vi "TLB Native Dynamic Events ver 0.09.vi"() -> ()   [LabVIEW 2018]
uses:
  Labview Training Phase 2/Enum Controls/States for Action Engine.ctl
  Type def/TLB event states.ctl
  Type def/TLB MHL States.ctl
  <vilib>/Studica/Studica Toolkit/Background/I2C Channel.ctl
  <vilib>/myRIO/Common/Instrument Driver Framework/myRIO v1.0/AI/typedefs/AI Channels Enum.ctl
  <vilib>/myRIO/Common/Instrument Driver Framework/myRIO v1.0/AI/typedefs/AI Channels List.ctl
  Type def/Type def.ctl
  <vilib>/addons/control/pid/NI_PID_pid.lvlib
  Underlying VI's/Webcam FGV Low level ver/State control.ctl
  <vilib>/userdefined/High Color/IMAQdx.ctl
  <vilib>/Studica/Studica Toolkit/NavX/NavX.lvlib
  <vilib>/addons/control/pid/pid.llb/PID (DBL).vi
  Underlying VI's/Movement control (archived)/Motor Control/States for motor control.ctl
  <vilib>/NI_Real-Time Target Support.lvlib
panel:
  out "Arduino Data":T1
  in  "STOP TASK":bool
  out "Waveform Chart 2":dbl(graph)
  in  "Select task":i8
  in  "OK Button":bool
  out "Yaw":dbl
  out "Speed and distance cluster":T2
  out "Decision":i8
  in  "STOP":bool
  out "error out":errorcluster
  out "Object detection count":T3
  out "Camera error":errorcluster
  out "element":T4
  out "Action Queue Items":i32
  out "State Logic Queue Items":i32
  out "Action Queues items":string[](array[string])=["Hardware reset", "Software reset", ""]
  out "State logic":T5=enum."Task 2"
  out "Action State":string
  # "TLB FRAMEWORK STATUS"
  # "Camera Status Loop"
  # "Test Programme written by Calvin Loke    Dated: 28 Aug 2019\nTest Programme revised by Dr Alex See   Dated 30 Aug 2019\n\nProgramme version:   TLB Native Dynamic Events ver 0.04b.vi"
  # "Motor Control Loop"
  # "NAVX Control Loop"
  # "Blackhawk status"
  # "System Health Status Update"
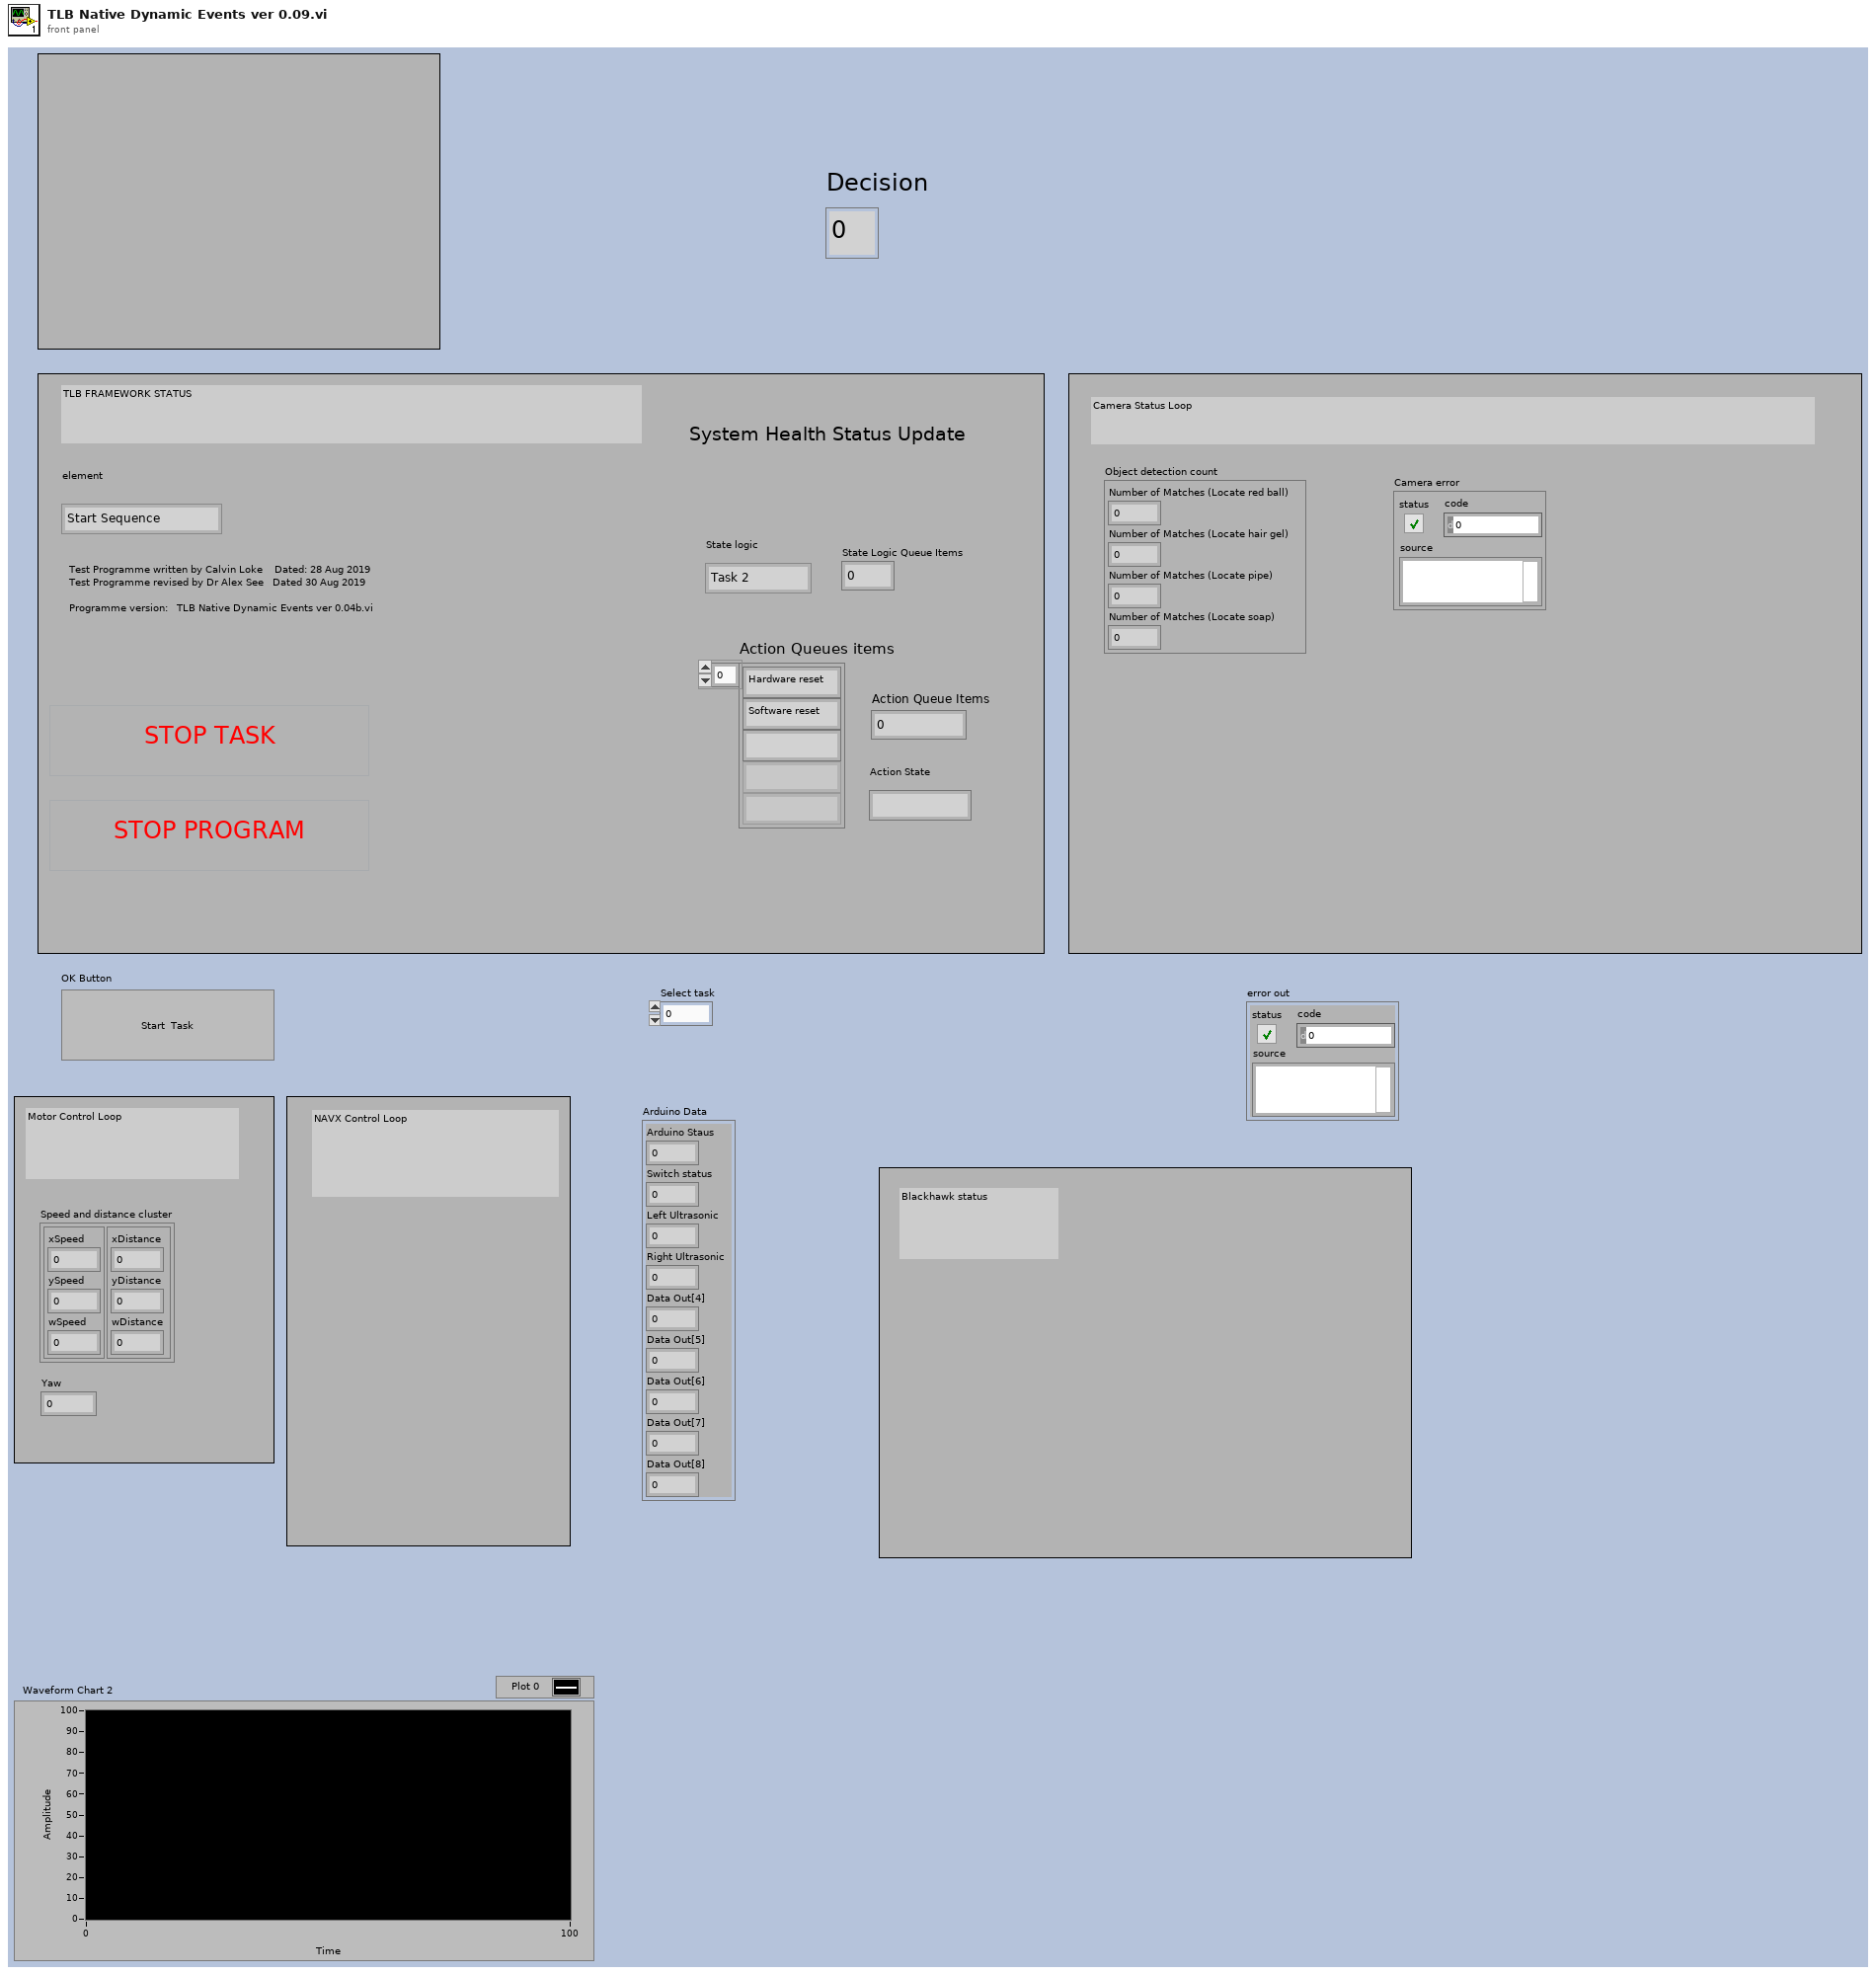
[diagram p1: front panel]
types:
  T1 = cluster{"Arduino Staus":u8, "Switch status":u8, "Left Ultrasonic":u8, "Right Ultrasonic":u8, "Data Out[4]":u8, "Data Out[5]":u8, "Data Out[6]":u8, "Data Out[7]":u8, "Data Out[8]":u8}
  T2 = cluster{cluster{"xSpeed":dbl, "ySpeed":dbl, "wSpeed":dbl}, cluster{"xDistance":dbl, "yDistance":dbl, "wDistance":dbl}}
  T3 = cluster{"Number of Matches (Locate red ball)":i32, "Number of Matches (Locate hair gel)":i32, "Number of Matches (Locate pipe)":i32, "Number of Matches (Locate soap)":i32}
  T4 = typedef "TLB event states.ctl" = enum16{"Start Sequence", "Exit", "Start Task 1", "Start Task 2", "Start Task 3", "Start Task 4", "Camera vision", "Wall follow mode", "Idle", "Start Drive Straight"}
  T5 = typedef "TLB MHL States.ctl" = enum16{"None", "Startup", "Idle", "Processing", "Shutdown", "Reset", "Task 1", "Task 2", "Task 3", "Task 4", "Task 4a", "Task 4b", "Task 4c", "Task 4d", "Task 4e", "Task 4f", "Task 4g", "Task 4h", "Acquire image", "Wall follow mode", "Autodrive", "Autodrive a"}
  T6 = typedef "States for motor control.ctl" = enum16{"LAST STATE", "STOP", "FORWARD", "BACKWARD", "LEFT", "RIGHT", "RCW", "ACW", "INIT", "RESET ENCODERS"}
  T7 = typedef "States for Action Engine.ctl" = enum16{"Initialize", "Write", "Read"}
  T8 = typedef "Type def.ctl" = cluster{"Front Ultrasonic Obstruct":bool, "Left Ultrasonic Obstruct":bool, "Right Ultrasonic Obstruct ":bool}
  T9 = typedef "I2C Channel.ctl" = enum16{"Not Connected", "A", "B"}
  T10 = enum16{"LAST STATE", "STOP", "FORWARD", "BACKWARD", "LEFT", "RIGHT", "RCW", "ACW", "INIT", "RESET ENCODERS"}
  T11 = cluster{"proportional gain (Kc)":dbl, "integral time (Ti, min)":dbl, "derivative time (Td, min)":dbl}
  T12 = typedef "State control.ctl" = enum16{"Initialise", "Start camera", "Continuous Acquisition ", "Stop camera", "Dispose all"}
  T13 = typedef "IMAQdx.ctl" = refnum<k21>
  T14 = cluster{"Arduino Status":u8, "Task Selection":u8, "PING_A":u8, "PING_B":u8, "PING_C":u8, "PING_D":u8, "Compass Low Byte":u8, "Compass High Byte":u8, "Data Out[8]":u8}
  T15 = typedef "AI Channels List.ctl" = T16[]
  T16 = typedef "AI Channels Enum.ctl" = enum16{"Not Connected", "AudioIn/Left", "AudioIn/Right", "C/AI0", "C/AI1", "A/AI0", "A/AI1", "A/AI2", "A/AI3", "A/AI4", "A/AI5", "A/AI6", "A/AI7", "B/AI0", "B/AI1", "B/AI2", "B/AI3", "B/AI4", "B/AI5", "B/AI6", "B/AI7", "AI/AI0", "AI/AI1", "AI/AI2", "AI/AI3", "A/AI0 (DIFF)", "A/AI1 (DIFF)", "A/AI2 (DIFF)", "A/AI3 (DIFF)", "B/AI0 (DIFF)", "B/AI1 (DIFF)", "B/AI2 (DIFF)", "B/AI3 (DIFF)"}
  T17 = typedef "NI_Real-Time Target Support.lvlib/RT CPU Load.ctl" = cluster{"Total (%)":dbl, "Time Critical (%)":dbl, "Timed Structures (%)":dbl, "High (%)":dbl, "Above Normal (%)":dbl, "Normal (%)":dbl, "Background (%)":dbl, "Idle (%)":dbl, "ISR (%)":dbl}
  T18 = cluster{"I2C Ref Out":cluster{"I2C Channel":T9, "FPGA VI Reference Out":refnum<k20>}, "Connected":bool, "Slave Address (7-bit)":u8, "Registry":u8[]}
  T19 = typedef "IMAQ Image.ctl" = refnum<image>
  T20 = cluster{"CPU loads[0]":T17, "CPU loads[1]":T17, "CPU loads[2]":T17, "CPU loads[3]":T17, "CPU loads[4]":T17, "CPU loads[5]":T17, "CPU loads[6]":T17, "CPU loads[7]":T17, "CPU loads[8]":T17}
  T21 = cluster{"Yaw":dbl, "Roll":dbl, "Pitch":dbl, "Heading":dbl, "Fused Heading":dbl}
  T22 = cluster{"xDistance":dbl, "yDistance":dbl, "wDistance":dbl}
  T23 = cluster{"I2C Channel":T9, "FPGA VI Reference Out":refnum<k20>}
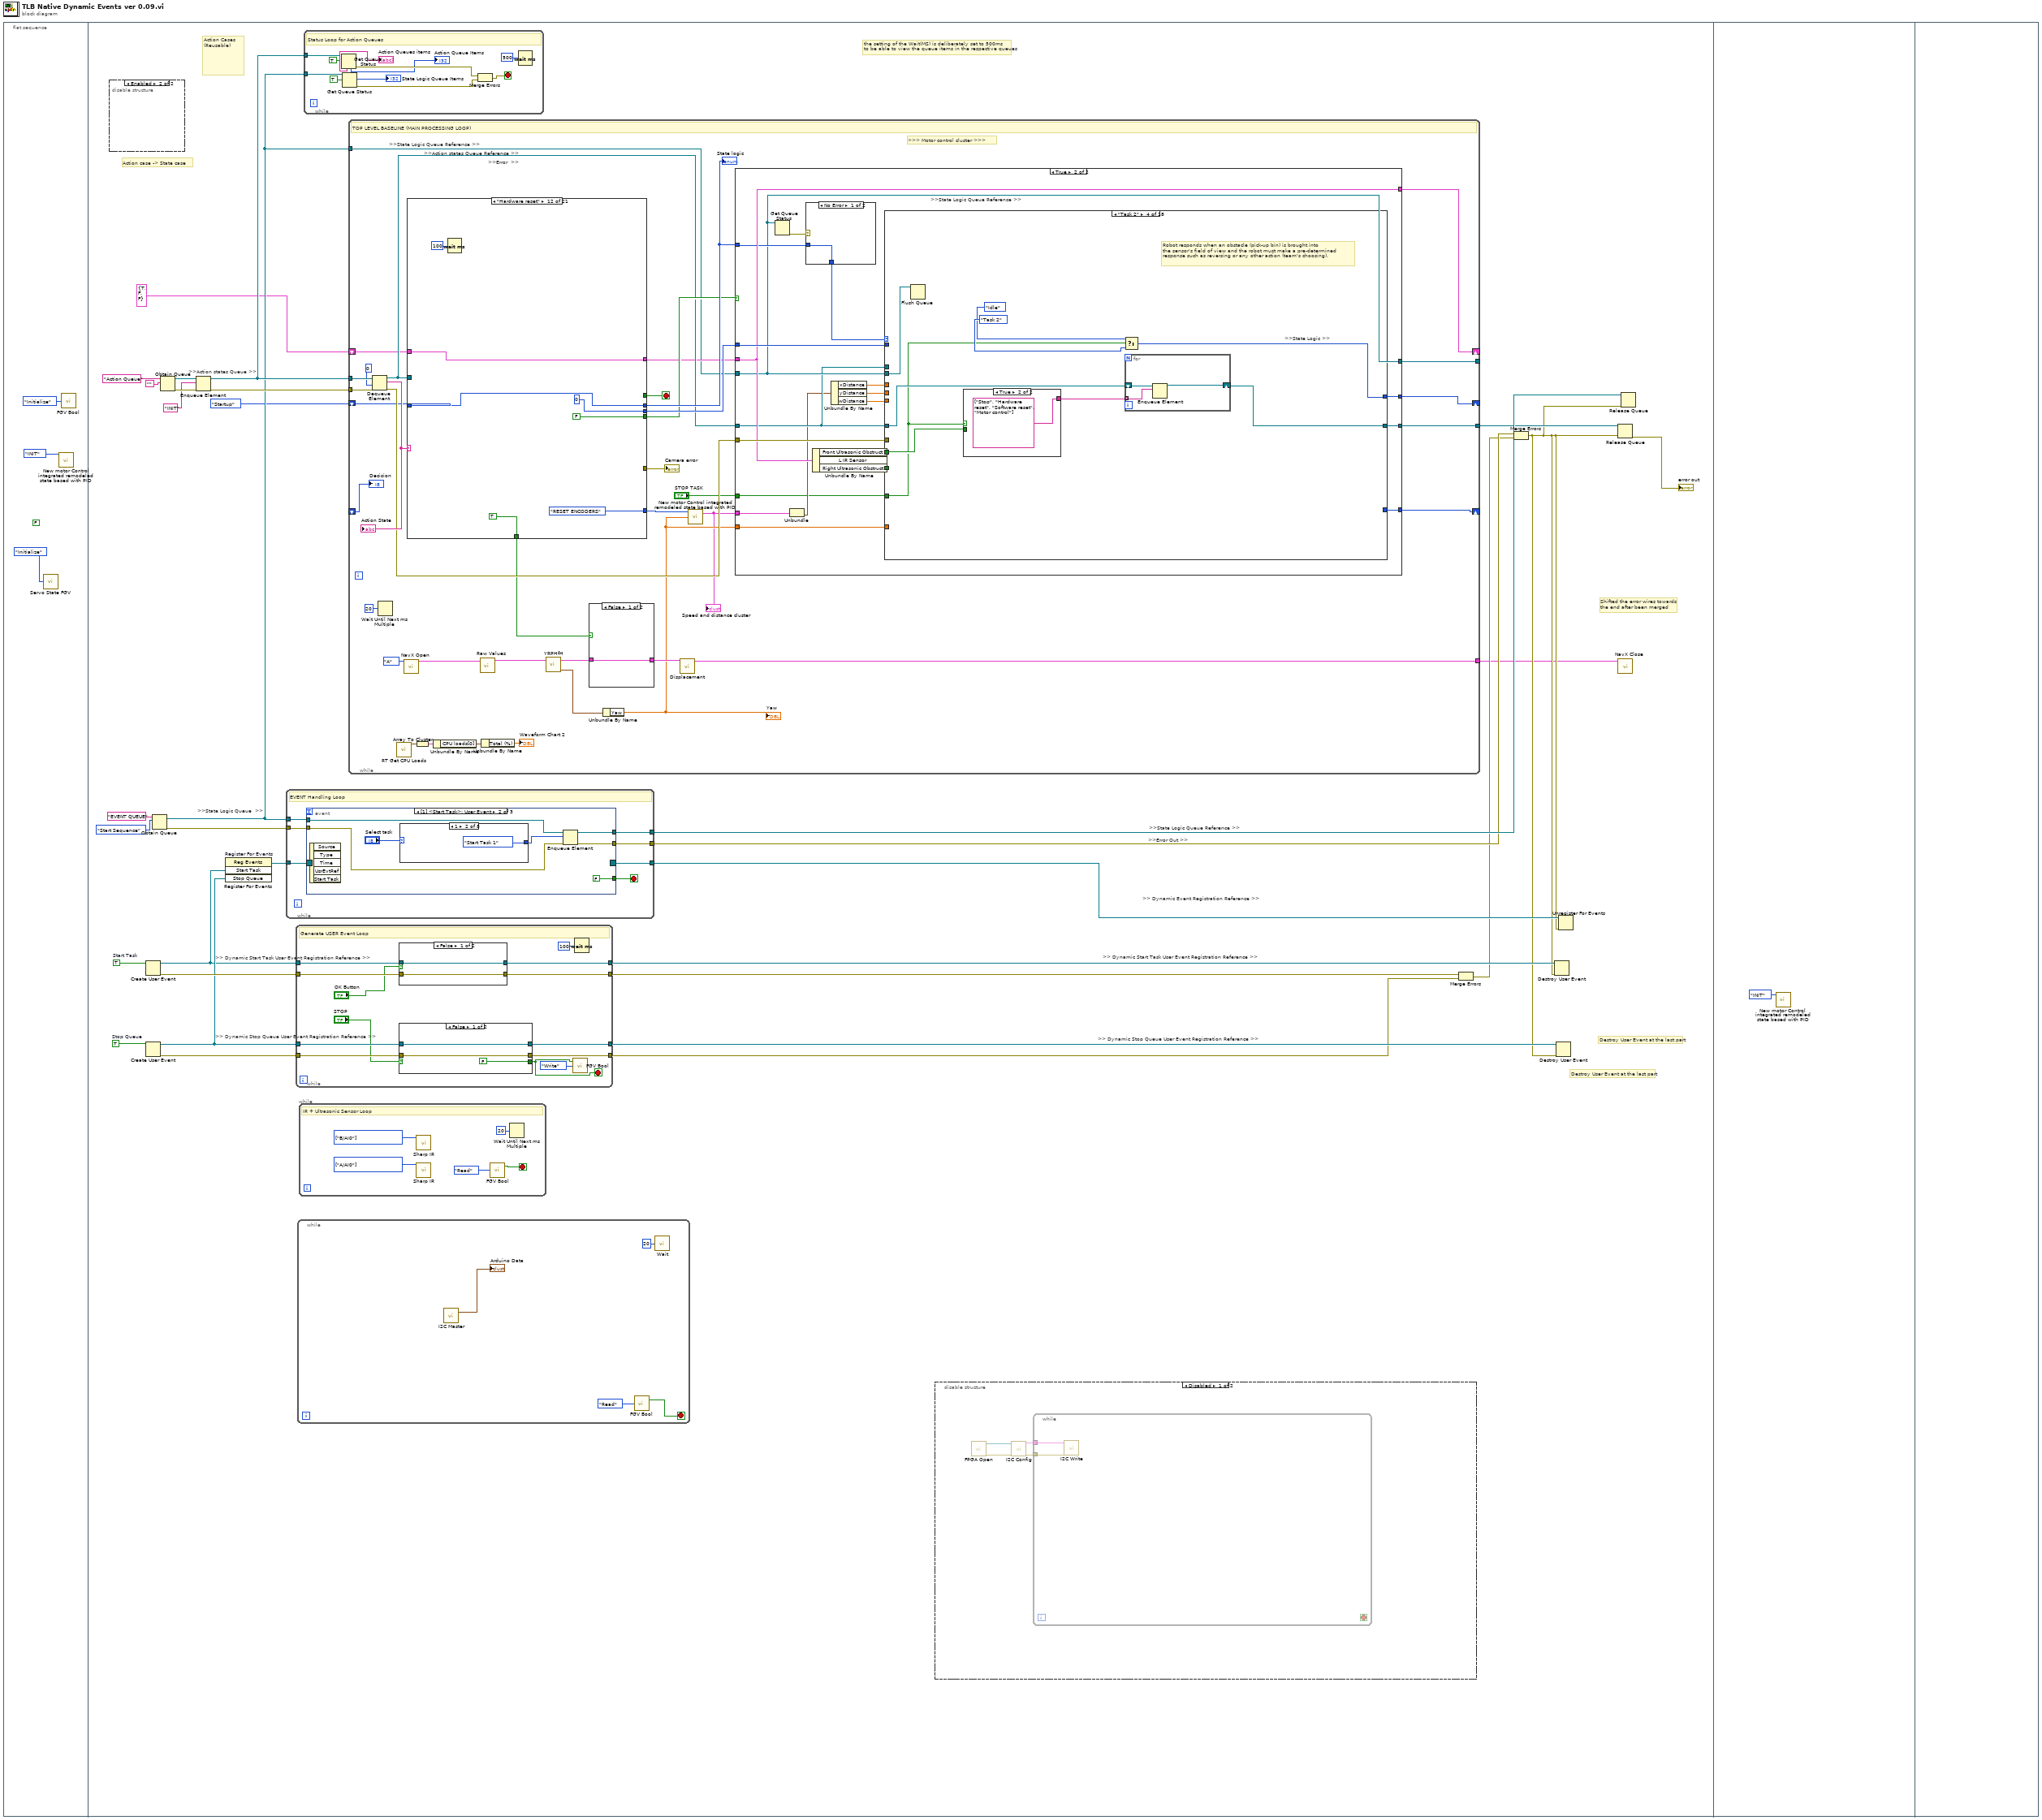
[diagram p0: block diagram]
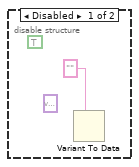
[diagram p3: hidden frame]
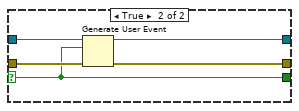
[diagram p4: hidden frame]
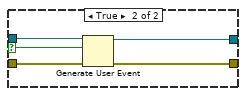
[diagram p5: hidden frame]
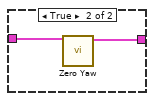
[diagram p6: hidden frame]
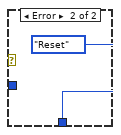
[diagram p8: hidden frame]
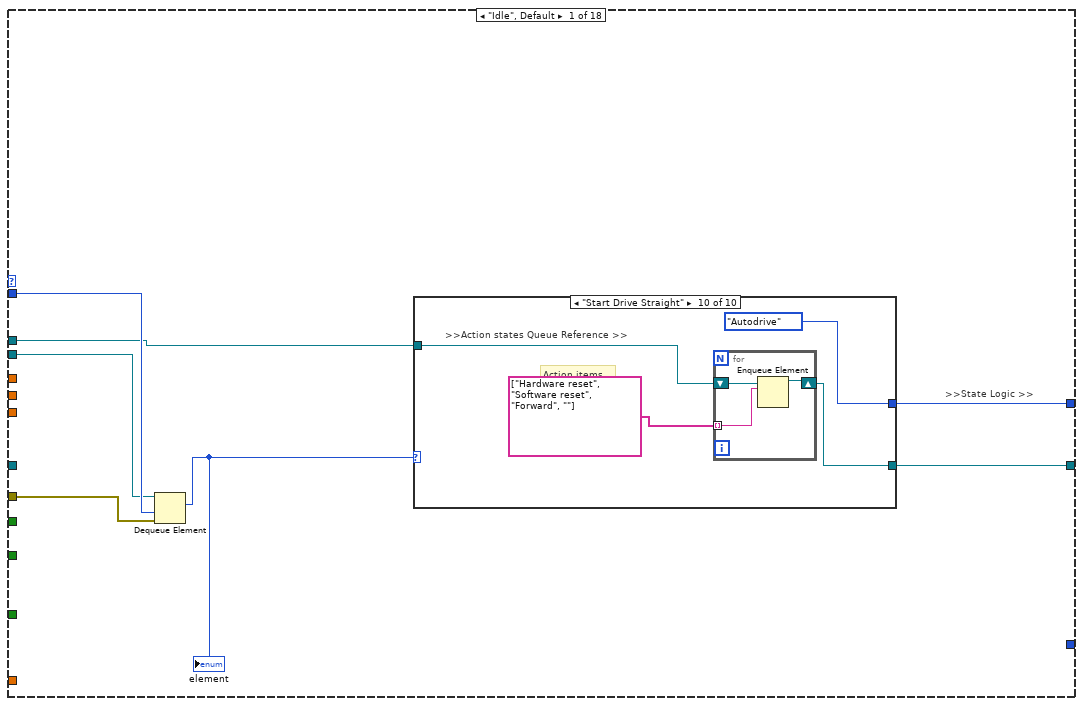
[diagram p9: hidden frame]
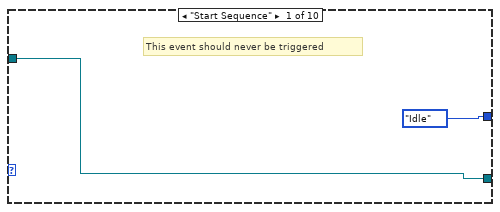
[diagram p10: hidden frame]
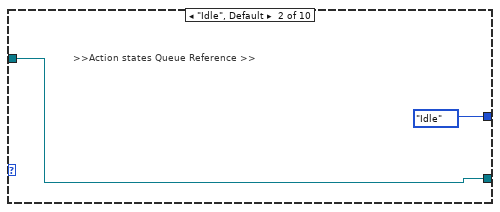
[diagram p11: hidden frame]
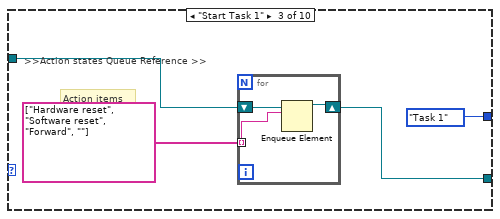
[diagram p12: hidden frame]
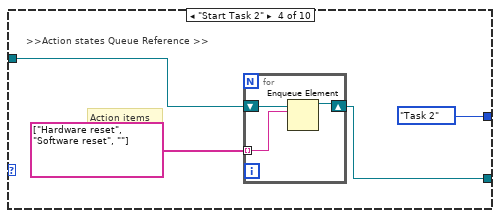
[diagram p13: hidden frame]
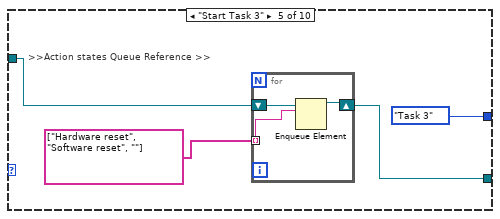
[diagram p14: hidden frame]
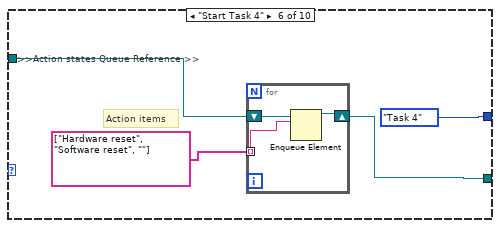
[diagram p15: hidden frame]
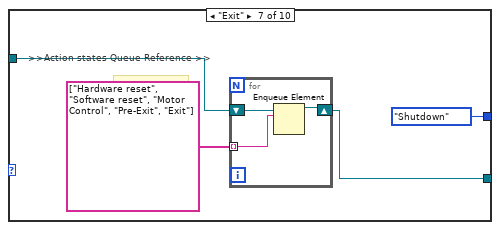
[diagram p16: hidden frame]
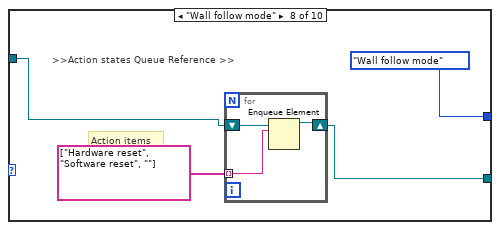
[diagram p17: hidden frame]
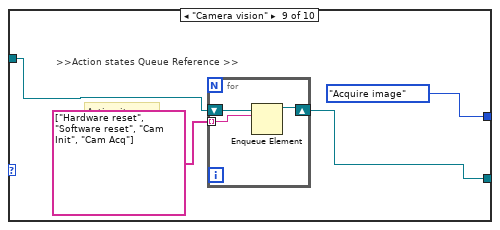
[diagram p18: hidden frame]
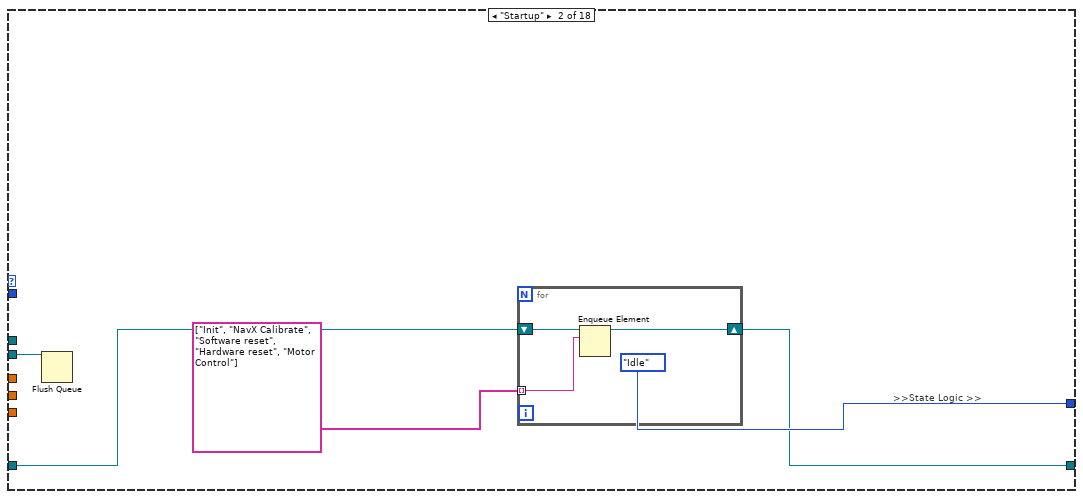
[diagram p19: hidden frame]
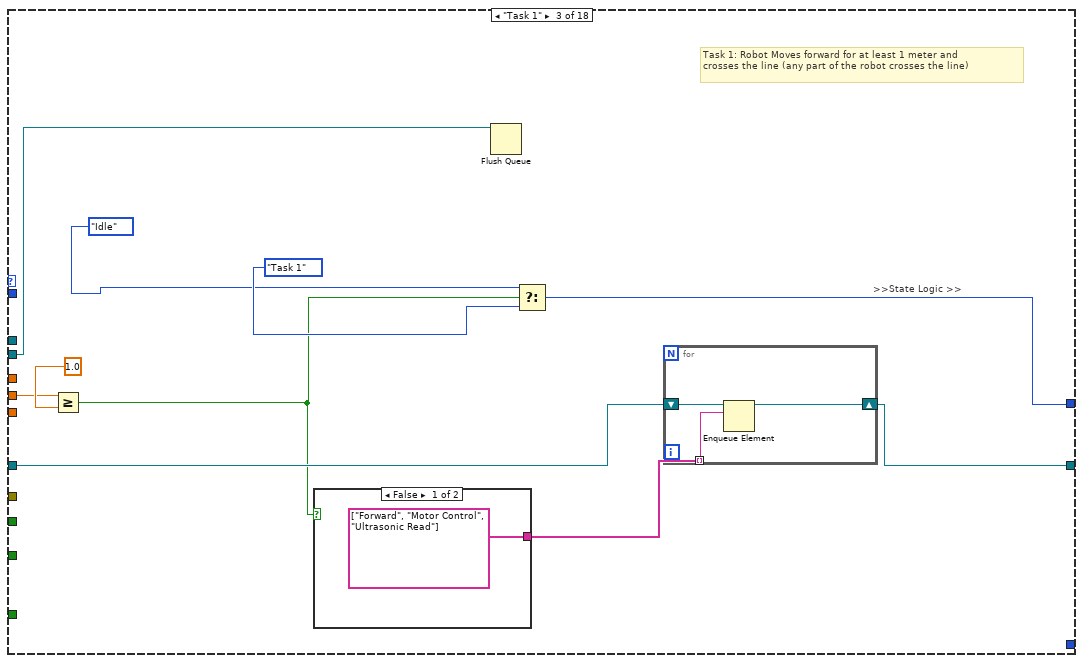
[diagram p20: hidden frame]
diagram:
  n1 = flat-sequence {
    frame #0 {
      (unwired) FALSE ("DIO 1")
      n2 = call "Servo State FGV.vi"("Init/Read/Write State"=States_for_Action_Engine."Initialize") -> ()  [unwired: 2 in, 2 out]
      n3 = call "New motor Control integrated remodeled state based with PID.vi"("States"=States_for_motor_control."INIT") -> ()  [unwired: 2 in, 2 out]
      n4 = call "FGV Bool.vi"("Init/Read/Write State"=States_for_Action_Engine."Initialize") -> ()  [unwired: 2 in, 2 out]
    }
    frame #1 {
      w35 = TRUE  # Stop Queue
      w34 = TRUE  # Start Task
      # "Action case -> State case"
      # "the setting of the Wait(MS) is deliberately set to 500ms\nto be able to view the queue items in the respective queues"
      # "Action Cases\n(Reusable)"
      # ">>Error Out >>"
      # ">> Dynamic Stop Queue User Event Registration Reference >>"
      # ">> Dynamic Start Task User Event Registration Reference >>"
      # ">> Dynamic Stop Queue User Event Registration Reference >>"
      # ">> Dynamic Start Task User Event Registration Reference >>"
      # ">> Dynamic Event Registration Reference >>"
      # ">>Action states Queue >>"
      # ">>State Logic Queue  >>"
      # ">>State Logic Queue Reference >>"
      # "Destroy User Event at the last part"
      # "Destroy User Event at the last part"
      # "Shifted the error wires towards\nthe end after been merged"
      n5 = disable-structure shown="Enabled" {
        frame Disabled {
          (unwired) variant
          (unwired) TRUE
          n6 = Variant To Data(type="") -> ()  [unwired: 2 in, 2 out]
        }
        frame Enabled {
        }
      }
      n7 = Create User Event(user event datatype=w34) -> (user event=w26:refnum<user-event>, error out=w31:errorcluster)  [unwired: 1 in]
      n8 = Create User Event(user event datatype=w35) -> (user event=w27:refnum<user-event>, error out=w30:errorcluster)  [unwired: 1 in]
      n9 = Obtain Queue(name (unnamed)="EVENT QUEUE", element data type=TLB_event_states."Start Sequence" ("Enum")) -> (queue out=w11:refnum<queue>, error out=w17:errorcluster)  [unwired: 3 in, 1 out]
      n10 = Obtain Queue(name (unnamed)="Action Queue", element data type="") -> (queue out=w20:refnum<queue>, error out=w16:errorcluster)  [unwired: 3 in, 1 out]
      n11 = Enqueue Element(queue=w20, element="INIT", error in (no error)=w16) -> (queue out=w12:refnum<queue>, error out=w15:errorcluster)  [unwired: 1 in, 1 out]
      n12 = register-events "Register For Events"(w26, w27) -> (reference out=w25:refnum<event-registration>)  [unwired: 2 in, 1 out]
      n13 = while {
        tunnel: w25 -> [w592]
        tunnel: [w591] -> w24
        tunnel: w11 -> [w589]
        tunnel: [w588] -> w23
        tunnel: w17 -> [w587]
        tunnel: [w586] -> w14
        stop <- w590 stop-if-true
        # "EVENT Handling Loop"
        n14 = event shown="[1] <Start Task>: User Event" {
          selector: w592 -> [_ _ _]
          dyn-events: [_ _ _] -> w591
          timeout: _ -> [_ _ _]
          tunnel: [FALSE FALSE w619] -> w590
          tunnel: w589 -> [w597 w604 w617]
          tunnel: [w596 w603 w618] -> w588
          tunnel: w587 -> [w594 w602 w615]
          tunnel: [w593 w601 w614] -> w586
          event Timeout {
            n15 = event-data() -> ()  [unwired: 1 in, 3 out]
            n16 = Enqueue Element(queue=w597, element=TLB_event_states."Idle" ("Enum"), error in (no error)=w594) -> (queue out=w596:refnum<queue>, error out=w593:errorcluster)  [unwired: 1 in, 1 out]
          }
          event User Event {
            n17 = event-data() -> ()  [unwired: 1 in, 5 out]
            n18 = case shown="1" "Select task" {
              tunnel: [TLB_event_states."Idle" ("Enum") TLB_event_states."Start Task 1" ("Enum") TLB_event_states."Start Task 2" ("Enum") TLB_event_states."Start Task 3" ("Enum") TLB_event_states."Start Task 4" ("Enum") TLB_event_states."Wall follow mode" ("Enum") TLB_event_states."Camera vision" ("Enum") TLB_event_states."Start Drive Straight" ("Enum")] -> w600
              frame 0 {
              }
              frame 1 {
              }
              frame 2 {
              }
              frame 3, Default {
              }
              frame 4 {
              }
              frame 5 {
              }
              frame 6 {
              }
              frame 7 {
              }
            }
            n19 = Enqueue Element(queue=w604, element=w600, error in (no error)=w602) -> (queue out=w603:refnum<queue>, error out=w601:errorcluster)  [unwired: 1 in, 1 out]
          }
          event User Event {
            n20 = event-data() -> ("Stop Queue"=w619:bool)  [unwired: 1 in, 4 out]
            n21 = Enqueue Element At Opposite End(queue=w617, element=TLB_event_states."Exit" ("Enum"), error in (no error)=w615) -> (queue out=w618:refnum<queue>, error out=w614:errorcluster)  [unwired: 1 in, 1 out]
          }
        }
      }
      n22 = while {
        tunnel: w26 -> [w69]
        tunnel: w27 -> [w68]
        tunnel: [w67] -> w33
        tunnel: [w66] -> w32
        tunnel: w31 -> [w65]
        tunnel: [w64] -> w29
        tunnel: w30 -> [w63]
        tunnel: [w62] -> w28
        stop <- w60 stop-if-true
        # "Generate USER Event Loop"
        n23 = case shown="False" "OK Button" {
          selector: "OK Button" -> [_ w81]
          tunnel: w69 -> [w80 w85]
          tunnel: [w80 w84] -> w66
          tunnel: w65 -> [w79 w83]
          tunnel: [w79 w82] -> w64
          frame False {
          }
          frame True {
            n24 = Generate User Event(user event=w85, event data cluster=w81, error in=w83) -> (user event out=w84:refnum<user-event>, error out=w82:errorcluster)  [unwired: 1 in]
          }
        }
        n25 = case shown="False" "STOP" {
          selector: "STOP" -> [_ w74]
          tunnel: w68 -> [w73 w78]
          tunnel: [w73 w77] -> w67
          tunnel: w63 -> [w72 w76]
          tunnel: [w72 w75] -> w62
          tunnel: [FALSE w74] -> w60
          frame False {
          }
          frame True {
            n26 = Generate User Event(user event=w78, event data cluster=w74, error in=w76) -> (user event out=w77:refnum<user-event>, error out=w75:errorcluster)  [unwired: 1 in]
          }
        }
        n27 = call "FGV Bool.vi"("Init/Read/Write State"=States_for_Action_Engine."Write", "Input Node"=w60) -> ()  [unwired: 1 in, 2 out]
        n28 = Wait (ms)(milliseconds to wait=u32 100) -> ()  [unwired: 1 out]
      }
      n29 = while {
        stop <- w38 stop-if-true
        n30 = call "I2C Master.vi"() -> ("Arduino Data"=→"Arduino Data":T14)  [unwired: 2 in, 1 out]
        n31 = call "FGV Bool.vi"("Init/Read/Write State"=States_for_Action_Engine."Read") -> ("Output node"=w38:bool)  [unwired: 2 in, 1 out]
        n32 = call "Wait"("Count(uSec)"=u32 20) -> ()  [unwired: 1 out]
      }
      n33 = while {
        stop <- w581 stop-if-true
        w584 = T15 [enum."A/AI0"] items=["Not Connected", "AudioIn/Left", "AudioIn/Right", "C/AI0", "C/AI1", "A/AI0", "A/AI1", "A/AI2", "A/AI3", "A/AI4", "A/AI5", "A/AI6", "A/AI7", "B/AI0", "B/AI1", "B/AI2", "B/AI3", "B/AI4", "B/AI5", "B/AI6", "B/AI7", "AI/AI0", "AI/AI1", "AI/AI2", "AI/AI3", "A/AI0 (DIFF)", "A/AI1 (DIFF)", "A/AI2 (DIFF)", "A/AI3 (DIFF)", "B/AI0 (DIFF)", "B/AI1 (DIFF)", "B/AI2 (DIFF)", "B/AI3 (DIFF)"] ("AI Channel")
        w585 = T15 [enum."B/AI0"] items=["Not Connected", "AudioIn/Left", "AudioIn/Right", "C/AI0", "C/AI1", "A/AI0", "A/AI1", "A/AI2", "A/AI3", "A/AI4", "A/AI5", "A/AI6", "A/AI7", "B/AI0", "B/AI1", "B/AI2", "B/AI3", "B/AI4", "B/AI5", "B/AI6", "B/AI7", "AI/AI0", "AI/AI1", "AI/AI2", "AI/AI3", "A/AI0 (DIFF)", "A/AI1 (DIFF)", "A/AI2 (DIFF)", "A/AI3 (DIFF)", "B/AI0 (DIFF)", "B/AI1 (DIFF)", "B/AI2 (DIFF)", "B/AI3 (DIFF)"] ("AI Channel")
        # "IR + Ultrasonic Sensor Loop"
        n34 = call <vilib>:"Sharp IR.vi"("AI Channel"=w585) -> ()  [unwired: 8 in, 3 out]
        n35 = call <vilib>:"Sharp IR.vi"("AI Channel"=w584) -> ()  [unwired: 8 in, 3 out]
        n36 = call "FGV Bool.vi"("Init/Read/Write State"=States_for_Action_Engine."Read") -> ("Output node"=w581:bool)  [unwired: 2 in, 1 out]
        n37 = Wait Until Next ms Multiple(millisecond multiple=u32 20) -> ()  [unwired: 1 out]
      }
      n38 = while {
        tunnel: w12 -> [w55]
        tunnel: w11 -> [w52]
        stop <- w49 stop-if-true
        # "Status Loop for Action Queues"
        n39 = Get Queue Status(queue=w55, return elements? (F)=TRUE) -> (error out=w51:errorcluster, # elements in queue=→"Action Queue Items":i32, elements=→"Action Queues items":string[])  [unwired: 1 in, 5 out]
        n40 = Get Queue Status(queue=w52, return elements? (F)=TRUE) -> (# pending remove=→"State Logic Queue Items":i32, error out=w50:errorcluster)  [unwired: 1 in, 6 out]
        n41 = Merge Errors(w51, w50) -> (w49:errorcluster)
        n42 = Wait (ms)(milliseconds to wait=u32 500) -> ()  [unwired: 1 out]
      }
      n43 = while {
        tunnel: w11 -> [w106]
        shift-right: [w117] -> _
        shift-left: TLB_MHL_States."Startup" ("Enum") -> [w111]
        tunnel: w12 -> [w122]
        tunnel: w15 -> [w120]
        tunnel: [w119] -> _
        tunnel: [w118] -> w7
        shift-right: [w108] -> _
        shift-left: T8 {"Front Ultrasonic Obstruct"=TRUE, "Left Ultrasonic Obstruct"=FALSE, "Right Ultrasonic Obstruct "=FALSE} -> [w110]
        shift-right: [w103] -> _
        shift-left: _ -> [w102]
        tunnel: [w95] -> w4
        stop <- w104 stop-if-true
        # ">>> Motor control cluster >>>"
        # ">>Error  >>"
        # ">>Action states Queue Reference >>"
        # ">>State Logic Queue Reference >>"
        # "TOP LEVEL BASELINE (MAIN PROCESSING LOOP)"
        n44 = Dequeue Element(queue=w122, timeout in ms (-1)=0, error in (no error)=w120) -> (queue out=w112:refnum<queue>, element=w121:string, error out=w113:errorcluster)  [unwired: 1 out]
        "Action State" <- w121
        n45 = Wait Until Next ms Multiple(millisecond multiple=u32 20) -> ()  [unwired: 1 out]
        n46 = call <vilib>:"RT Get CPU Loads.vi"() -> ("CPU loads"=w87:T17[])  [unwired: 10 in, 1 out]
        n47 = call <vilib>:"NavX Open.vi"("I2C Channel"=I2C_Channel."A") -> ("NavX Info"=w97:T18)  [unwired: 9 in, 1 out]
        n48 = case shown="\"Hardware reset\"" w121 {
          tunnel: [w435 w449 w455 w460 w465 w471 w476 w479 w486 w491 w501 w508 TLB_MHL_States."Shutdown" ("Enum") w518 w532 w536 w546 w556 w564 w575 w579] -> w123
          tunnel: [w438 0 0 0 0 0 0 0 0 0 0 0 0 0 0 0 0 0 0 0 0] -> w116
          tunnel: [TRUE FALSE FALSE FALSE FALSE FALSE FALSE FALSE FALSE FALSE FALSE FALSE FALSE FALSE FALSE FALSE FALSE FALSE FALSE FALSE FALSE] -> w115
          tunnel: w112 -> [_ _ _ _ _ _ _ _ _ _ _ _ _ _ _ _ _ _ _ _ _]
          tunnel: w111 -> [w435 w449 w455 w460 w465 w471 w476 w479 w486 w491 w501 w508 _ w518 w532 w536 w546 w556 w564 w575 w579]
          tunnel: w110 -> [w436 w445 w452 w461 w463 w468 w473 w478 w483 w489 w498 w505 w511 w519 w531 w538 w547 w557 w563 w572 w580]
          tunnel: [w436 w444 w451 w461 w463 w468 w473 w478 w483 w489 w497 w505 w511 w519 w528 w537 w547 w557 w563 w572 w580] -> w109
          tunnel: [_ _ _ _ _ _ _ _ _ _ _ _ _ _ _ _ _ w548 w559 w567 _] -> w107
          tunnel: [_ _ _ _ _ _ _ _ _ _ _ _ TRUE _ _ _ _ _ _ _ _] -> w104
          tunnel: [T10."LAST STATE" ("Move mode") T10."INIT" ("Move mode") T10."FORWARD" ("Move mode") T10."LAST STATE" ("Move mode") T10."BACKWARD" ("Move mode") T10."RIGHT" ("Move mode") T10."LEFT" ("Move mode") T10."RCW" ("Move mode") T10."ACW" ("Move mode") T10."STOP" ("Move mode") _ T10."RESET ENCODERS" ("Move mode") T10."INIT" ("Move mode") T10."INIT" ("Move mode") _ _ _ _ _ _ _] -> w93
          tunnel: [FALSE ("NavX Zero Yaw") _ _ _ _ _ _ _ _ FALSE ("NavX Zero Yaw") FALSE ("NavX Zero Yaw") TRUE ("NavX Zero Yaw") _ _ _ _ _ _ _ _ _] -> w94
          frame "No action", Default {
            n49 = case shown="\"Startup\", Default" w435 {
              tunnel: [0 100] -> w438
              frame "Startup", Default {
              }
              frame "Idle" {
              }
            }
          }
          frame "Init" {
            # ">>State Logic  >>"
            n50 = Bundle By Name(cluster=w445, "Front Ultrasonic Obstruct"=FALSE ("Object detected"), "L IR Sensor"=0.0, "Right Ultrasonic Obstruct"=FALSE ("In move state?")) -> (w444:T8)
          }
          frame "Forward" {
            n51 = Bundle By Name(cluster=w452, "Right Ultrasonic Obstruct"=TRUE ("In move state?")) -> (w451:T8)
          }
          frame " Motor Control" {
          }
          frame "Reverse" {
          }
          frame "Right" {
          }
          frame "Left" {
          }
          frame "Rotate CW" {
          }
          frame "Rotate ACW" {
          }
          frame "Stop" {
          }
          frame "Software reset" {
            w493 = FALSE ("In move state?")
            # "Resets any software variables\nand/or non-critical states"
            n52 = Wait (ms)(milliseconds to wait=u32 20) -> ()  [unwired: 1 out]
            n53 = Bundle By Name(cluster=w498, "Front Ultrasonic Obstruct"=w493, "L IR Sensor"=0.0, "Right Ultrasonic Obstruct"=w493) -> (w497:T8)
          }
          frame "Hardware reset" {
            n54 = Wait (ms)(milliseconds to wait=u32 100) -> ()  [unwired: 1 out]
          }
          frame "Exit" {
          }
          frame "Pre-Exit" {
          }
          frame "Ultrasonic read" {
            # "Object detection"
            n55 = local read "Arduino Data"() -> (w527:T1)
            n56 = Unbundle By Name(w527) -> ("Left Ultrasonic"=w525:u8, "Right Ultrasonic"=w526:u8)
            n57 = Add(x=w525, y=w526) -> (x+y=w524:u8)
            n58 = Divide(x=w524, y=u8 2) -> (x/y=w522:dbl)
            n59 = Less?(x=w522, y=20.0) -> (x < y?=w520:bool)
            n60 = Bundle By Name(cluster=w531, "Front Ultrasonic Obstruct"=w520) -> (w528:T8)
          }
          frame "IR Sensor Read" {
            n61 = Bundle By Name(cluster=w538, "L IR Sensor"=0.0) -> (w537:T8)
          }
          frame "Calculate" {
            n62 = Unbundle By Name(w547) -> ("L IR Sensor"=w542:dbl)
            n63 = call-poly <vilib>:"PID.vi"("output range"=cluster{"output high":dbl, "output low":dbl} {"output high"=0.3, "output low"=-0.3}, "PID gains"=T11 {"proportional gain (Kc)"=0.01, "integral time (Ti, min)"=0.0, "derivative time (Td, min)"=0.0}, "process variable"=w542, "setpoint"=20.0) -> ("output"=w539:dbl)  [unwired: 6 in, 1 out]
            n64 = Negate(x=w539) -> ()  [unwired: 1 out]
          }
          frame "Cam Init" {
            n65 = call "Low-Level Grab.vi"("States"=State_control."Initialise", "Session In"=T13 "cam1") -> ("error out"=w549:errorcluster, "Session Out"=w550:T13)  [unwired: 7 in, 1 out]
            n66 = call "Low-Level Grab.vi"("error in (no error)"=w549, "States"=State_control."Start camera", "Session In"=w550) -> ("error out"=w548:errorcluster)  [unwired: 6 in, 2 out]
          }
          frame "Cam Acq" {
            n67 = call "Low-Level Grab.vi"("States"=State_control."Continuous Acquisition ") -> ("error out"=w560:errorcluster, "Image Out"=w561:T19)  [unwired: 8 in, 1 out]
            n68 = call "All object detection ver2.vi"("Image In"=w561, "error in"=w560) -> ("Object detection count"=→"Object detection count":T3, "error out"=w559:errorcluster)  [unwired: 1 out]
          }
          frame "Cam Exit" {
            n69 = call "Low-Level Grab.vi"("States"=State_control."Stop camera") -> ("error out"=w568:errorcluster, "Session Out"=w570:T13)  [unwired: 8 in, 1 out]
            n70 = call "Low-Level Grab.vi"("error in (no error)"=w568, "States"=State_control."Dispose all", "Session In"=w570) -> ("error out"=w567:errorcluster)  [unwired: 6 in, 2 out]
          }
          frame "NavX Calibrate" {
            # "Adds a 15 second delay to the startup process \nfor the NavX to calibrate"
            n71 = Wait (ms)(milliseconds to wait=u32 2000) -> ()  [unwired: 1 out]
          }
        }
        "State logic" <- w123
        "Camera error" <- w107
        n72 = Array To Cluster(array=w87) -> (cluster=w88:T20)
        n73 = Unbundle By Name(w88) -> ("CPU loads[0]"=w89:T17)
        n74 = call <vilib>:"Raw Values.vi"("NavX Info In"=w97) -> ("NavX Info Out"=w100:T18)  [unwired: 8 in, 1 out]
        n75 = Unbundle By Name(w89) -> ("Total (%)"=→"Waveform Chart 2":dbl)
        n76 = call <vilib>:"YRPHfH.vi"("NavX Info In"=w100) -> ("YRPHfH"=w101:T21, "NavX Info Out"=w99:T18)  [unwired: 3 in]
        n77 = case shown="False" w94 {
          tunnel: [w124 w126] -> w96
          tunnel: w99 -> [w124 w125]
          frame False {
          }
          frame True {
            n78 = call <vilib>:"Zero Yaw.vi"("NavX Info In"=w125) -> ("NavX Info Out"=w126:T18)  [unwired: 10 in]
          }
        }
        n79 = Unbundle By Name(w101) -> ("Yaw"=w92:dbl)
        "Yaw" <- w92
        n80 = call <vilib>:"Displacement.vi"("NavX Info In"=w96) -> ("NavX Info Out"=w95:T18)  [unwired: 9 in, 1 out]
        n81 = call "New motor Control integrated remodeled state based with PID.vi"("Yaw"=w92, "States"=w93) -> ("Speed and distance cluster"=w91:T2)  [unwired: 1 in, 1 out]
        "Speed and distance cluster" <- w91
        n82 = case shown="True" w115 {
          tunnel: w123 -> [w129 w140]
          tunnel: w106 -> [w130 w139]
          tunnel: w112 -> [w128 w137]
          tunnel: [w130 w139] -> w119
          tunnel: [w128 w150] -> w118
          tunnel: [w129 w149] -> w117
          tunnel: w113 -> [_ w148]
          tunnel: w116 -> [_ w147]
          tunnel: w109 -> [w127 w142]
          tunnel: [w127 w142] -> w108
          tunnel: w91 -> [_ w135]
          tunnel: [_ w133] -> w103
          tunnel: w92 -> [_ w132]
          tunnel: "STOP TASK" -> [_ w131]
          frame False {
          }
          frame True {
            # ">>State Logic Queue Reference >>"
            n83 = Get Queue Status(queue=w139) -> (error out=w138:errorcluster)  [unwired: 2 in, 7 out]
            n84 = Unbundle(w135) -> (w134:T22)  [unwired: 1 out]
            n85 = case shown="No Error" w138 {
              tunnel: [w151 TLB_MHL_States."Reset" ("Enum")] -> w141
              tunnel: w140 -> [w151 _]
              frame No Error {
              }
              frame Error {
              }
            }
            n86 = Unbundle By Name(w142) -> ("Front Ultrasonic Obstruct"=w143:bool, "Right Ultrasonic Obstruct"=w136:bool)  [unwired: 1 out]
            n87 = Unbundle By Name(w134) -> ("xDistance"=w144:dbl, "yDistance"=w146:dbl, "wDistance"=w145:dbl)
            n88 = case shown="\"Task 2\"" w141 {
              tunnel: w139 -> [w155 w220 w229 w244 w263 w277 w291 w306 w321 w336 _ w358 w378 w391 _ _ _ _]
              tunnel: w137 -> [_ w222 w233 w247 w270 w280 w295 w311 w325 w341 w351 w360 w379 w394 w403 w406 w412 w426]
              tunnel: [w153 w221 w232 w248 w269 w281 w294 w310 w324 w340 w350 w361 w380 w393 w403 w405 w412 w427] -> w150
              tunnel: [w158 TLB_MHL_States."Idle" ("Enum") w235 w249 w266 w284 w297 w309 w326 w339 TLB_MHL_States."Shutdown" ("Enum") w363 w373 w392 TLB_MHL_States."Reset" ("Enum") TLB_MHL_States."Shutdown" ("Enum") TLB_MHL_States."Reset" ("Enum") w423] -> w149
              tunnel: w148 -> [w156 _ _ _ _ _ _ _ _ _ _ _ _ _ _ _ _ _]
              tunnel: w147 -> [w157 _ _ _ _ _ _ _ _ _ _ _ _ _ _ _ _ _]
              tunnel: w146 -> [_ _ w228 _ _ _ w290 w305 _ _ _ _ _ _ _ _ _ _]
              tunnel: w145 -> [_ _ _ _ w261 _ _ _ _ _ _ _ _ _ _ _ _ _]
              tunnel: w144 -> [_ _ _ _ _ _ _ _ w320 _ _ _ _ _ _ _ _ _]
              tunnel: w143 -> [_ _ _ w245 _ w278 _ _ _ w338 _ _ w375 w390 _ _ _ _]
              tunnel: w137 -> [w154 _ _ _ _ _ _ _ _ _ _ _ _ _ _ _ _ _]
              tunnel: w136 -> [_ _ _ _ _ _ _ _ _ _ _ _ _ _ _ _ _ _]
              tunnel: [_ _ _ _ _ _ _ _ _ _ _ _ w371 _ _ _ _ _] -> w133
              tunnel: w132 -> [_ _ _ _ _ _ _ _ _ _ _ _ _ _ _ _ _ w415]
              tunnel: w131 -> [_ _ _ w243 w260 _ _ _ _ w335 _ w357 w370 _ _ _ _ w414]
              frame "Idle", Default {
                # ">>State Logic >>"
                n89 = Dequeue Element(queue=w155, timeout in ms (-1)=w157, error in (no error)=w156) -> (element=w159:T4)  [unwired: 3 out]
                "element" <- w159
                n90 = case shown="\"Start Drive Straight\"" w159 {
                  tunnel: [TLB_MHL_States."Idle" ("Enum") TLB_MHL_States."Idle" ("Enum") TLB_MHL_States."Task 1" ("Enum") TLB_MHL_States."Task 2" ("Enum") TLB_MHL_States."Task 3" ("Enum") TLB_MHL_States."Task 4" ("Enum") TLB_MHL_States."Shutdown" ("Enum") TLB_MHL_States."Wall follow mode" ("Enum") TLB_MHL_States."Acquire image" ("Enum") TLB_MHL_States."Autodrive" ("Enum")] -> w158
                  tunnel: w154 -> [w160 w162 w166 w173 w179 w187 w194 w201 w208 w215]
                  tunnel: [w160 w162 w165 w172 w180 w186 w193 w200 w207 w213] -> w153
                  frame "Start Sequence" {
                    # "This event should never be triggered"
                  }
                  frame "Idle", Default {
                    # ">>Action states Queue Reference >>"
                  }
                  frame "Start Task 1" {
                    # ">>Action states Queue Reference >>"
                    # "Action items"
                    n91 = for {
                      shift-right: [w170] -> w165
                      shift-left: w166 -> [w169]
                      tunnel: string[] ["Hardware reset", "Software reset", "Forward", ""] -> [w168] mode=indexing
                      n92 = Enqueue Element(queue=w169, element=w168) -> (queue out=w170:refnum<queue>)  [unwired: 2 in, 2 out]
                    }
                  }
                  frame "Start Task 2" {
                    # ">>Action states Queue Reference >>"
                    # "Action items"
                    n93 = for {
                      shift-right: [w177] -> w172
                      shift-left: w173 -> [w176]
                      tunnel: string[] ["Hardware reset", "Software reset", ""] -> [w175] mode=indexing
                      n94 = Enqueue Element(queue=w176, element=w175) -> (queue out=w177:refnum<queue>)  [unwired: 2 in, 2 out]
                    }
                  }
                  frame "Start Task 3" {
                    # ">>Action states Queue Reference >>"
                    n95 = for {
                      shift-right: [w184] -> w180
                      shift-left: w179 -> [w183]
                      tunnel: string[] ["Hardware reset", "Software reset", ""] -> [w182] mode=indexing
                      n96 = Enqueue Element(queue=w183, element=w182) -> (queue out=w184:refnum<queue>)  [unwired: 2 in, 2 out]
                    }
                  }
                  frame "Start Task 4" {
                    # ">>Action states Queue Reference >>"
                    # "Action items"
                    n97 = for {
                      shift-right: [w191] -> w186
                      shift-left: w187 -> [w190]
                      tunnel: string[] ["Hardware reset", "Software reset", ""] -> [w189] mode=indexing
                      n98 = Enqueue Element(queue=w190, element=w189) -> (queue out=w191:refnum<queue>)  [unwired: 2 in, 2 out]
                    }
                  }
                  frame "Exit" {
                    # ">>Action states Queue Reference >>"
                    # "Action items"
                    n99 = for {
                      shift-right: [w198] -> w193
                      shift-left: w194 -> [w197]
                      tunnel: string[] ["Hardware reset", "Software reset", "Motor Control", "Pre-Exit", "Exit"] -> [w196] mode=indexing
                      n100 = Enqueue Element(queue=w197, element=w196) -> (queue out=w198:refnum<queue>)  [unwired: 2 in, 2 out]
                    }
                  }
                  frame "Wall follow mode" {
                    # ">>Action states Queue Reference >>"
                    # "Action items"
                    n101 = for {
                      shift-right: [w205] -> w200
                      shift-left: w201 -> [w204]
                      tunnel: string[] ["Hardware reset", "Software reset", ""] -> [w203] mode=indexing
                      n102 = Enqueue Element(queue=w204, element=w203) -> (queue out=w205:refnum<queue>)  [unwired: 2 in, 2 out]
                    }
                  }
                  frame "Camera vision" {
                    # ">>Action states Queue Reference >>"
                    # "Action items"
                    n103 = for {
                      shift-right: [w212] -> w207
                      shift-left: w208 -> [w211]
                      tunnel: string[] ["Hardware reset", "Software reset", "Cam Init", "Cam Acq"] -> [w210] mode=indexing
                      n104 = Enqueue Element(queue=w211, element=w210) -> (queue out=w212:refnum<queue>)  [unwired: 2 in, 2 out]
                    }
                  }
                  frame "Start Drive Straight" {
                    # ">>Action states Queue Reference >>"
                    # "Action items"
                    n105 = for {
                      shift-right: [w219] -> w213
                      shift-left: w215 -> [w218]
                      tunnel: string[] ["Hardware reset", "Software reset", "Forward", ""] -> [w217] mode=indexing
                      n106 = Enqueue Element(queue=w218, element=w217) -> (queue out=w219:refnum<queue>)  [unwired: 2 in, 2 out]
                    }
                  }
                }
              }
              frame "Startup" {
                # ">>State Logic >>"
                n107 = Flush Queue(queue=w220) -> ()  [unwired: 1 in, 3 out]
                n108 = for {
                  shift-right: [w226] -> w221
                  shift-left: w222 -> [w227]
                  tunnel: string[] ["Init", "NavX Calibrate", "Software reset", "Hardware reset", "Motor Control"] -> [w225] mode=indexing
                  n109 = Enqueue Element(queue=w227, element=w225) -> (queue out=w226:refnum<queue>)  [unwired: 2 in, 2 out]
                }
              }
              frame "Task 1" {
                # "Task 1: Robot Moves forward for at least 1 meter and\ncrosses the line (any part of the robot crosses the line)"
                # ">>State Logic >>"
                n110 = Greater Or Equal?(x=w228, y=1.0) -> (x >= y?=w230:bool)
                n111 = case shown="False" w230 {
                  tunnel: [string[] ["Forward", "Motor Control", "Ultrasonic Read"] string[] ["Software reset", "Hardware reset", "Motor Control"]] -> w234
                  frame False {
                  }
                  frame True {
                  }
                }
                n112 = Flush Queue(queue=w229) -> ()  [unwired: 1 in, 3 out]
                n113 = Select(t=TLB_MHL_States."Idle" ("Enum"), s=w230, f=TLB_MHL_States."Task 1" ("Enum")) -> (s? t:f=w235:T5)
                n114 = for {
                  shift-right: [w241] -> w232
                  shift-left: w233 -> [w242]
                  tunnel: w234 -> [w240] mode=indexing
                  n115 = Enqueue Element(queue=w242, element=w240) -> (queue out=w241:refnum<queue>)  [unwired: 2 in, 2 out]
                }
              }
              frame "Task 2" {
                # "Robot responds when an obstacle (pick-up bin) is brought into\nthe sensor's field of view and the robot must make a pre-determined \nresponse such as reversing or any other action (team's choosing)."
                # ">>State Logic >>"
                n116 = Flush Queue(queue=w244) -> ()  [unwired: 1 in, 3 out]
                n117 = case shown="True" w243 {
                  tunnel: [w253 string[] ["Stop", "Hardware reset", "Software reset", "Motor control"]] -> w246
                  tunnel: w245 -> [w252 _]
                  frame False {
                    n118 = case shown="False" w252 {
                      tunnel: [string[] ["Stop", "Ultrasonic read", "Motor Control"] string[] ["Reverse", "Ultrasonic read", "Motor control"]] -> w253
                      frame False {
                      }
                      frame True {
                      }
                    }
                  }
                  frame True {
                  }
                }
                n119 = Select(t=TLB_MHL_States."Idle" ("Enum"), s=w243, f=TLB_MHL_States."Task 2" ("Enum")) -> (s? t:f=w249:T5)
                n120 = for {
                  shift-right: [w258] -> w248
                  shift-left: w247 -> [w259]
                  tunnel: w246 -> [w257] mode=indexing
                  n121 = Enqueue Element(queue=w259, element=w257) -> (queue out=w258:refnum<queue>)  [unwired: 2 in, 2 out]
                }
              }
              frame "Task 3" {
                # "Robot rotates at least 360 degrees within a 0.42m by a 0.3m space\n(footprint of robot's base must always be within the 0.42m x 0.3m\nboundary at all times during the rotation)."
                n122 = Greater Or Equal?(x=w261, y=360.0) -> (x >= y?=w264:bool)
                n123 = Flush Queue(queue=w263) -> ()  [unwired: 1 in, 3 out]
                n124 = Or(x=w264, y=w260) -> (x .or. y?=w265:bool)
                n125 = case shown="False" w265 {
                  tunnel: [string[] ["Rotate CW", "Motor Control"] string[] ["Software reset", "Hardware reset", "Motor Control"]] -> w271
                  frame False {
                  }
                  frame True {
                  }
                }
                n126 = for {
                  shift-right: [w273] -> w269
                  shift-left: w270 -> [w274]
                  tunnel: w271 -> [w272] mode=indexing
                  n127 = Enqueue Element(queue=w274, element=w272) -> (queue out=w273:refnum<queue>)  [unwired: 2 in, 2 out]
                }
                n128 = Select(t=TLB_MHL_States."Idle" ("Enum"), s=w265, f=TLB_MHL_States."Task 3" ("Enum")) -> (s? t:f=w266:T5)
              }
              frame "Task 4" {
                n129 = Flush Queue(queue=w277) -> ()  [unwired: 1 in, 3 out]
                n130 = case shown="True" w278 {
                  tunnel: [string[] ["Forward", "Ultrasonic read", "Motor Control"] string[] ["Stop", "Hardware reset", "Software reset", "Motor Control"]] -> w279
                  frame False {
                  }
                  frame True {
                  }
                }
                n131 = for {
                  shift-right: [w288] -> w281
                  shift-left: w280 -> [w289]
                  tunnel: w279 -> [w287] mode=indexing
                  n132 = Enqueue Element(queue=w289, element=w287) -> (queue out=w288:refnum<queue>)  [unwired: 2 in, 2 out]
                }
                n133 = Select(t=TLB_MHL_States."Task 4a" ("Enum"), s=w278, f=TLB_MHL_States."Task 4" ("Enum")) -> (s? t:f=w284:T5)
              }
              frame "Task 4a" {
                n134 = Greater Or Equal?(x=w290, y=0.5) -> (x >= y?=w293:bool)
                n135 = Flush Queue(queue=w291) -> ()  [unwired: 1 in, 3 out]
                n136 = case shown="True" w293 {
                  tunnel: [string[] ["Right", "Motor Control"] string[] ["Stop", "Hardware reset", "Software reset", "Motor Control"]] -> w296
                  frame False {
                  }
                  frame True {
                  }
                }
                n137 = for {
                  shift-right: [w303] -> w294
                  shift-left: w295 -> [w304]
                  tunnel: w296 -> [w302] mode=indexing
                  n138 = Enqueue Element(queue=w304, element=w302) -> (queue out=w303:refnum<queue>)  [unwired: 2 in, 2 out]
                }
                n139 = Select(t=TLB_MHL_States."Task 4b" ("Enum"), s=w293, f=TLB_MHL_States."Task 4a" ("Enum")) -> (s? t:f=w297:T5)
              }
              frame "Task 4b" {
                n140 = Flush Queue(queue=w306) -> ()  [unwired: 1 in, 3 out]
                n141 = Greater Or Equal?(x=w305, y=0.75) -> (x >= y?=w307:bool)
                n142 = case shown="False" w307 {
                  tunnel: [string[] ["Forward", "Motor control"] string[] ["Stop", "Hardware reset", "Software reset"]] -> w312
                  frame False {
                  }
                  frame True {
                  }
                }
                n143 = for {
                  shift-right: [w318] -> w310
                  shift-left: w311 -> [w319]
                  tunnel: w312 -> [w317] mode=indexing
                  n144 = Enqueue Element(queue=w319, element=w317) -> (queue out=w318:refnum<queue>)  [unwired: 2 in, 2 out]
                }
                n145 = Select(t=TLB_MHL_States."Task 4c" ("Enum"), s=w307, f=TLB_MHL_States."Task 4b" ("Enum")) -> (s? t:f=w309:T5)
              }
              frame "Task 4c" {
                n146 = Flush Queue(queue=w321) -> ()  [unwired: 1 in, 3 out]
                n147 = Less Or Equal?(x=w320, y=-0.65) -> (x <= y?=w322:bool)
                n148 = case shown="False" w322 {
                  tunnel: [string[] ["Left", "Motor Control"] string[] ["Stop", "Hardware reset", "Software reset", "Motor Control"]] -> w327
                  frame False {
                  }
                  frame True {
                  }
                }
                n149 = for {
                  shift-right: [w333] -> w324
                  shift-left: w325 -> [w334]
                  tunnel: w327 -> [w332] mode=indexing
                  n150 = Enqueue Element(queue=w334, element=w332) -> (queue out=w333:refnum<queue>)  [unwired: 2 in, 2 out]
                }
                n151 = Select(t=TLB_MHL_States."Task 4d" ("Enum"), s=w322, f=TLB_MHL_States."Task 4c" ("Enum")) -> (s? t:f=w326:T5)
              }
              frame "Task 4d" {
                n152 = Flush Queue(queue=w336) -> ()  [unwired: 1 in, 3 out]
                n153 = Or(x=w335, y=w338) -> (x .or. y?=w337:bool)
                n154 = case shown="True" w337 {
                  tunnel: [string[] ["Forward", "Ultrasonic Read", "Motor Control"] string[] ["Stop", "Hardware reset", "Software reset", "Motor Control"]] -> w342
                  frame False {
                  }
                  frame True {
                  }
                }
                n155 = for {
                  shift-right: [w348] -> w340
                  shift-left: w341 -> [w349]
                  tunnel: w342 -> [w347] mode=indexing
                  n156 = Enqueue Element(queue=w349, element=w347) -> (queue out=w348:refnum<queue>)  [unwired: 2 in, 2 out]
                }
                n157 = Select(t=TLB_MHL_States."Idle" ("Enum"), s=w337, f=TLB_MHL_States."Task 4d" ("Enum")) -> (s? t:f=w339:T5)
              }
              frame "Reset" {
                n158 = for {
                  shift-right: [w355] -> w350
                  shift-left: w351 -> [w356]
                  tunnel: string[] ["Software reset", "Hardware reset", "Motor Control"] -> [w354] mode=indexing
                  n159 = Enqueue Element(queue=w356, element=w354) -> (queue out=w355:refnum<queue>)  [unwired: 2 in, 2 out]
                }
              }
              frame "Wall follow mode" {
                n160 = Flush Queue(queue=w358) -> ()  [unwired: 1 in, 3 out]
                n161 = case shown="False" w357 {
                  tunnel: [string[] ["IR Sensor Read", "Calculate", "Forward", "Motor Control"] string[] ["Hardware reset", "Software reset", "Motor Control"]] -> w359
                  frame False {
                  }
                  frame True {
                  }
                }
                n162 = for {
                  shift-right: [w368] -> w361
                  shift-left: w360 -> [w369]
                  tunnel: w359 -> [w367] mode=indexing
                  n163 = Enqueue Element(queue=w369, element=w367) -> (queue out=w368:refnum<queue>)  [unwired: 2 in, 2 out]
                }
                n164 = Select(t=TLB_MHL_States."Idle" ("Enum"), s=w357, f=TLB_MHL_States."Wall follow mode" ("Enum")) -> (s? t:f=w363:T5)
              }
              frame "Autodrive" {
                # ">>>Return to idle event>>>"
                n165 = Flush Queue(queue=w378) -> ()  [unwired: 1 in, 3 out]
                n166 = Boolean To (0,1)(Boolean=w370) -> (0, 1=w377:i16)
                n167 = Boolean To (0,1)(Boolean=w375) -> (0, 1=w376:i16)
                n168 = formula code="int8  out;\nif (detect == 0 && stop == 0)\nout = 0;\n\nelse if (detect == 1 && stop == 0)\nout = 1;\n\nelse if (detect == 0 && stop == 1)\nout = 2;\n\nelse\nout = 0;"("stop"=w377, "detect"=w376) -> ("out"=w371:i8)
                n169 = case shown="2" w371 {
                  tunnel: [string[] ["Forward", "Ultrasonic read"] string[] ["Hardware reset", "Software reset", "Rotate Clockwise", ""] string[] ["Stop", "", "Software reset", "Motor Control"]] -> w374
                  frame 0, Default {
                  }
                  frame 1 {
                  }
                  frame 2 {
                  }
                }
                n170 = call "Servo State FGV.vi"("Init/Read/Write State"=States_for_Action_Engine."Write", "Servo State"=w371) -> ()  [unwired: 1 in, 2 out]
                n171 = for {
                  shift-right: [w388] -> w380
                  shift-left: w379 -> [w389]
                  tunnel: w374 -> [w387] mode=indexing
                  n172 = Enqueue Element(queue=w389, element=w387) -> (queue out=w388:refnum<queue>)  [unwired: 2 in, 2 out]
                }
                n173 = case shown="2" w371 {
                  tunnel: [TLB_MHL_States."Autodrive" ("Enum") TLB_MHL_States."Autodrive a" ("Enum") TLB_MHL_States."Idle" ("Enum")] -> w373
                  frame 0, Default {
                  }
                  frame 1 {
                  }
                  frame 2 {
                  }
                }
              }
              frame "Acquire image" {
                n174 = Flush Queue(queue=w391) -> ()  [unwired: 1 in, 3 out]
                n175 = case shown="False" w390 {
                  tunnel: [string[] ["Cam Acq"] string[] ["Hardware reset", "Software reset", "Cam Exit", ""]] -> w395
                  frame False {
                  }
                  frame True {
                  }
                }
                n176 = for {
                  shift-right: [w401] -> w393
                  shift-left: w394 -> [w402]
                  tunnel: w395 -> [w400] mode=indexing
                  n177 = Enqueue Element(queue=w402, element=w400) -> (queue out=w401:refnum<queue>)  [unwired: 2 in, 2 out]
                }
                n178 = Select(t=TLB_MHL_States."Idle" ("Enum"), s=w390, f=TLB_MHL_States."Acquire image" ("Enum")) -> (s? t:f=w392:T5)
              }
              frame "Processing" {
              }
              frame "Shutdown" {
                # ">>State Logic >>"
                n179 = for {
                  shift-right: [w410] -> w405
                  shift-left: w406 -> [w411]
                  tunnel: string[] ["Software reset", "Hardware reset", "Motor Control", "Cam Exit", "Pre-Exit", "Exit"] -> [w409] mode=indexing
                  n180 = Enqueue Element(queue=w411, element=w409) -> (queue out=w410:refnum<queue>)  [unwired: 2 in, 2 out]
                }
              }
              frame "None" {
              }
              frame "Autodrive a" {
                n181 = Greater Or Equal?(x=w415, y=80.0) -> (x >= y?=w416:bool)
                n182 = Or(x=w414, y=w416) -> (x .or. y?=w417:bool)
                n183 = case shown="True" w417 {
                  tunnel: [string[] ["Rotate CW", "Ultrasonic read", ""] string[] ["Stop", "", "Software reset", ""]] -> w425
                  frame False {
                  }
                  frame True {
                  }
                }
                n184 = for {
                  shift-right: [w431] -> w427
                  shift-left: w426 -> [w432]
                  tunnel: w425 -> [w430] mode=indexing
                  n185 = Enqueue Element(queue=w432, element=w430) -> (queue out=w431:refnum<queue>)  [unwired: 2 in, 2 out]
                }
                n186 = Or(x=w414, y=w416) -> (x .or. y?=w418:bool)
                n187 = Select(t=TLB_MHL_States."Idle" ("Enum"), s=w414, f=TLB_MHL_States."Autodrive" ("Enum")) -> (s? t:f=w421:T5)
                n188 = Select(t=w421, s=w418, f=TLB_MHL_States."Autodrive a" ("Enum")) -> (s? t:f=w423:T5)
              }
            }
          }
        }
        "Decision" <- w102
      }
      n189 = disable-structure shown="Disabled" {
        frame Disabled {
          n190 = call <vilib>:"FPGA Open.vi"() -> ("error out"=w43:errorcluster, "FPGA Reference Out"=w42:refnum<k20>)  [unwired: 10 in]
          n191 = call <vilib>:"I2C Config.vi"("error in (no error)"=w43, "FPGA Reference"=w42) -> ("error out"=w40:errorcluster, "I2C Ref Out"=w41:T23)  [unwired: 8 in]
          n192 = while {
            tunnel: w41 -> [w45]
            tunnel: w40 -> [w44]
            stop <- _ stop-if-true
            n193 = call <vilib>:"I2C Write.vi"("error in (no error)"=w44, "I2C Ref In"=w45) -> ()  [unwired: 8 in, 2 out]
          }
        }
        frame Enabled {
        }
      }
      n194 = Merge Errors "Merge Errors"(w29, w28) -> (w10:errorcluster)
      n195 = Merge Errors(w14, w10) -> (w5:errorcluster)
      n196 = Destroy User Event(user event=w32, error in=w5) -> ()  [unwired: 1 out]
      n197 = Destroy User Event(user event=w33, error in=w5) -> ()  [unwired: 1 out]
      n198 = Unregister For Events(event registration refnum=w24, error in=w5) -> ()  [unwired: 1 out]
      n199 = Release Queue(queue=w7, error in (no error)=w5) -> (error out=→"error out":errorcluster)  [unwired: 1 in, 2 out]
      n200 = call <vilib>:"NavX Close.vi"("NavX Info In"=w4) -> ()  [unwired: 10 in, 1 out]
      n201 = Release Queue(queue=w23, error in (no error)=w5) -> ()  [unwired: 1 in, 3 out]
    }
    frame #2 {
      n202 = call "New motor Control integrated remodeled state based with PID.vi"("States"=States_for_motor_control."INIT") -> ()  [unwired: 2 in, 2 out]
    }
    frame #3 {
    }
  }
